vi "ConfigureIncEncoderSensorType.vi"(4 "error in (no error)":errorcluster, 5 "SensorType":u16(ring)=1 items=["Incremental encoder with index (3-channel)", "Incremental encoder without index (2-channel)"], 6 "incremental encoder configuration":T1, 7 "axis in":cluster{"keyHandle":u32, "nodeId":u16}={"keyHandle"=0, "nodeId"=1}) -> (0 "error out":errorcluster, 3 "axis out":cluster{"keyHandle":u32, "nodeId":u16}={"keyHandle"=0, "nodeId"=1})   [LabVIEW 2017, in "maxonEPOS.lvlib"]
doc: "<B>ConfigureIncSensorType</B> writes the value for sensor type 'incremental encoder with index (3-channel)' to the device. Parameters from the sensor type can be set."
uses:
  Examples/maxonEPOS.lvlib
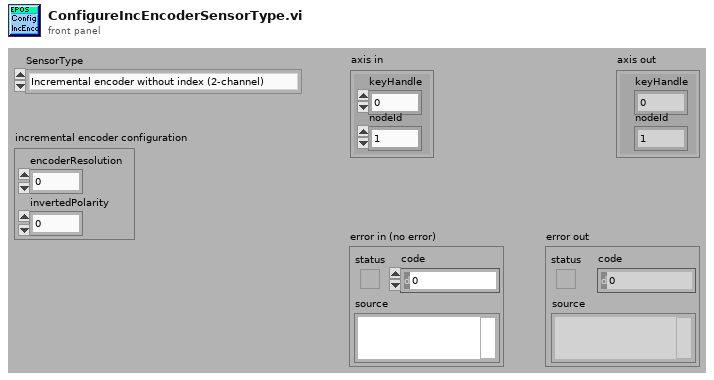
[diagram p1: front panel]
types:
  T1 = cluster{"encoderResolution":u32, "invertedPolarity":i32}
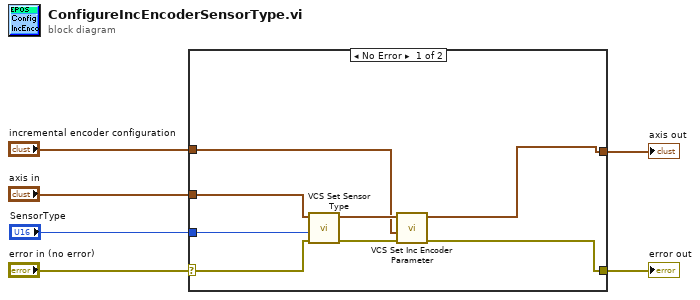
[diagram p0: block diagram]
diagram:
  n1 = case shown="No Error" "error in (no error)" {
    selector: "error in (no error)" -> [w13 w16]
    tunnel: [w8 w16] -> w5
    tunnel: [w9 w15] -> w4
    tunnel: "axis in" -> [w14 w15]
    tunnel: "incremental encoder configuration" -> [w10 _]
    tunnel: "SensorType" -> [w7 _]
    frame No Error {
      n2 = call "VCS Set Sensor Type.vi"("error in (no error)"=w13, "SensorType"=w7, "axis in"=w14) -> ("error out"=w12:errorcluster, "axis out"=w11:cluster{"keyHandle":u32, "nodeId":u16})  [unwired: 7 in]
      n3 = call "VCS Set Inc Encoder Parameter.vi"("error in (no error)"=w12, "Incremental encoder"=w10, "axis in"=w11) -> ("error out"=w8:errorcluster, "axis out"=w9:cluster{"keyHandle":u32, "nodeId":u16})  [unwired: 7 in]
    }
    frame Error {
    }
  }
  "error out" <- w5
  "axis out" <- w4
